vi "Read Error Status.vi"(8 "error in (no error)":errorcluster, 11 "VGC in":refnum<class "PL Inficon VGC.lvclass">) -> (0 "error out":errorcluster, 2 "error status":T1, 3 "VGC out":refnum<class "PL Inficon VGC.lvclass">)   [LabVIEW 2015, in "PL Inficon VGC.lvclass"]
doc: "Reads error status."
uses:
  PL Inficon VGC.lvclass
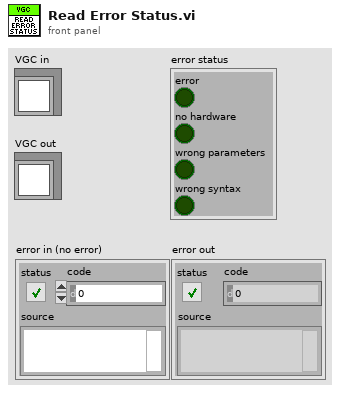
[diagram p1: front panel]
types:
  T1 = cluster{"error":bool, "no hardware":bool, "wrong parameters":bool, "wrong syntax":bool}
  T2 = cluster{"[0]":bool, "[1]":bool, "[2]":bool, "[3]":bool}
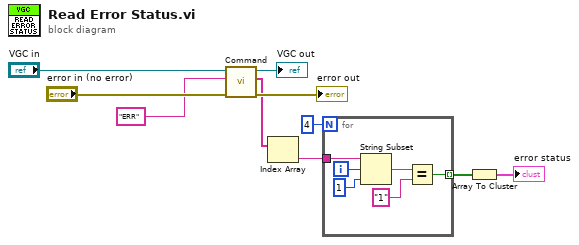
[diagram p0: block diagram]
diagram:
  n1 = call "Command.vi"("error in (no error)"="error in (no error)", "command"="ERR", "VGC in"="VGC in") -> ("error out"=→"error out":errorcluster, "response data"=w5:string[], "VGC out"=→"VGC out":refnum<class "PL Inficon VGC.lvclass">)  [unwired: 6 in]
  n2 = Index Array(array=w5) -> (element=w4:string)  [unwired: 1 in]
  n3 = for {
    N: 4 -> [_]
    tunnel: w4 -> [w16]
    tunnel: [w11] -> w2 mode=indexing
    i -> [w15]
    n4 = String Subset(string=w16, offset (0)=w15, length (rest)=1 ("length (rest)")) -> (substring=w13:string)
    n5 = Equal?(x=w13, y="1") -> (x = y?=w11:bool)
  }
  n6 = Array To Cluster(array=w2) -> (cluster=→"error status":T2)
